vi "Base Error Code.vi"() -> (3 "base error code":i32)   [LabVIEW 2017, in "UDP Transceiver.lvlib" / "UDP Transceiver.lvclass"]
uses:
  UDP Transceiver.lvclass
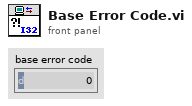
[diagram p1: front panel]
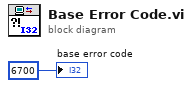
[diagram p0: block diagram]
diagram:
  "base error code" <- 6700 ("base error code")
